vi "Custom Config.vi"(8 "error in (no error)":errorcluster, 9 "Nikon Data":string, 11 "Nikon in":refnum<class "Nikon.lvclass">) -> (0 "error out":errorcluster, 3 "Nikon out":refnum<class "Nikon.lvclass">)   [LabVIEW 2021, in "Nikon.lvclass"]
uses:
  Nikon.lvclass
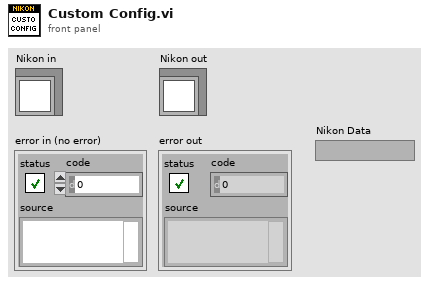
[diagram p1: front panel]
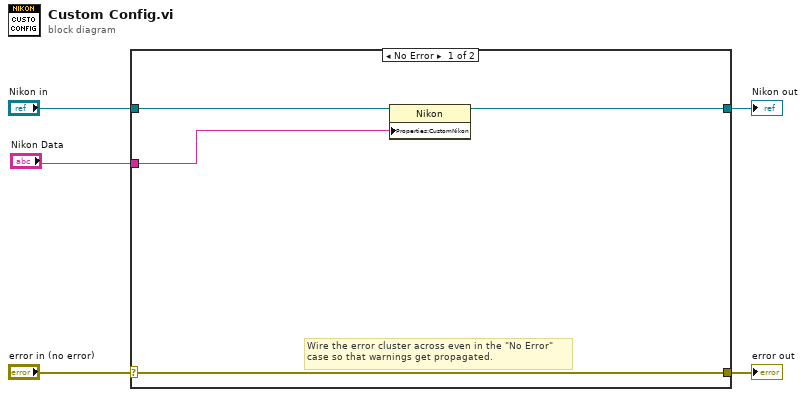
[diagram p0: block diagram]
diagram:
  n1 = case shown="No Error" "error in (no error)" {
    selector: "error in (no error)" -> [w8 w11]
    tunnel: [w8 w11] -> w4
    tunnel: [w7 w10] -> w2
    tunnel: "Nikon in" -> [w9 w10]
    tunnel: "Nikon Data" -> [w6 _]
    frame No Error {
      # "Wire the error cluster across even in the \"No Error\"\ncase so that warnings get propagated."
      n2 = property class="Nikon"(reference=w9, "Properties:CustomNikon"=w6) -> (reference out=w7:refnum<class "Nikon.lvclass">)  [unwired: 1 in, 1 out]
    }
    frame Error {
    }
  }
  "error out" <- w4
  "Nikon out" <- w2
